vi "Center Spin FR.vi"(0 "Wanted Angle":dbl, 1 "Current Angle":dbl) -> (7 "Motor Output":dbl format="%#_13g")   [LabVIEW 2020]
uses:
  <vilib>/addons/control/pid/pid.llb/PID (DBL).vi
  <vilib>/addons/control/pid/NI_PID_pid.lvlib
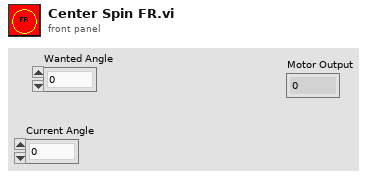
[diagram p1: front panel]
types:
  T1 = cluster{"proportional gain (Kc)":dbl, "integral time (Ti, min)":dbl, "derivative time (Td, min)":dbl}
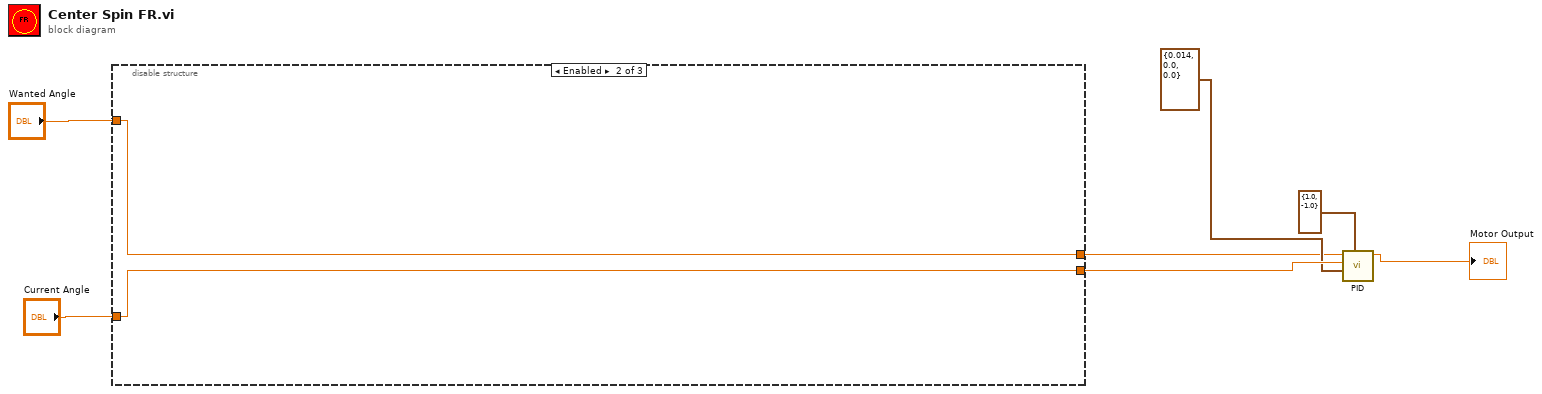
[diagram p0: block diagram]
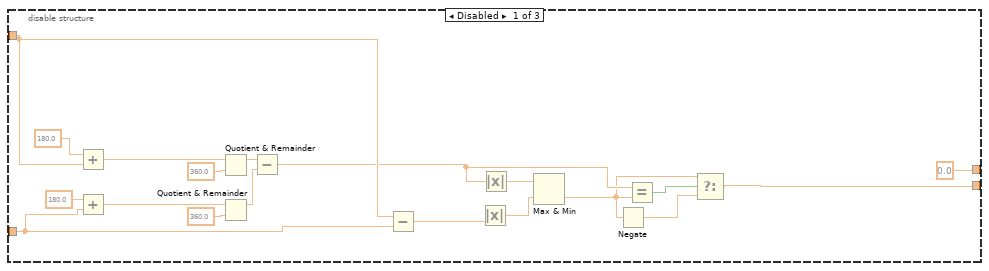
[diagram p2: hidden frame]
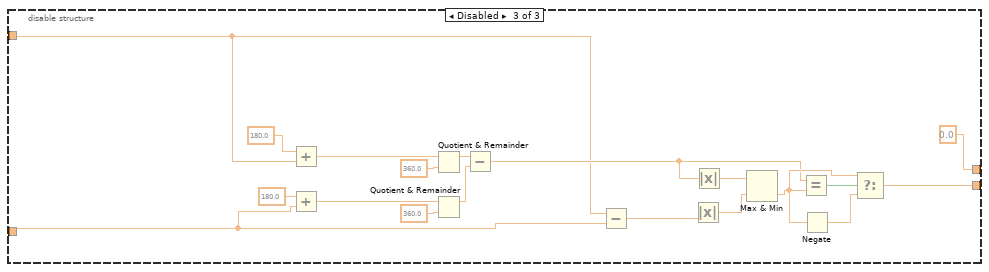
[diagram p3: hidden frame]
diagram:
  n1 = disable-structure shown="Enabled" {
    disable-tunnel: "Current Angle" -> [w26 w27 w31]
    disable-tunnel: "Wanted Angle" -> [w25 w28 w32]
    disable-tunnel: [w24 w27 w30] -> w4
    disable-tunnel: [0.0 w28 0.0] -> w1
    frame Disabled {
      n2 = Add(x=180.0, y=w25) -> (x+y=w10:dbl)
      n3 = Add(x=180.0, y=w26) -> (x+y=w11:dbl)
      n4 = Quotient & Remainder(x=w10, y=360.0) -> (x-y*floor(x/y)=w17:dbl)  [unwired: 1 out]
      n5 = Quotient & Remainder(x=w11, y=360.0) -> (x-y*floor(x/y)=w16:dbl)  [unwired: 1 out]
      n6 = Subtract(x=w17, y=w16) -> (x-y=w15:dbl)
      n7 = Subtract(x=w25, y=w26) -> (x-y=w18:dbl)
      n8 = Absolute Value(x=w18) -> (abs(x)=w12:dbl)
      n9 = Absolute Value(x=w15) -> (abs(x)=w9:dbl)
      n10 = Max & Min(x=w9, y=w12) -> (min(x,y)=w13:dbl)  [unwired: 1 out]
      n11 = Negate(x=w13) -> (-x=w14:dbl)
      n12 = Equal?(x=w15, y=w13) -> (x = y?=w23:bool)
      n13 = Select(t=w13, s=w23, f=w14) -> (s? t:f=w24:dbl)
    }
    frame Enabled {
    }
    frame Disabled {
      n14 = Add(x=180.0, y=w32) -> (x+y=w40:dbl)
      n15 = Add(x=180.0, y=w31) -> (x+y=w41:dbl)
      n16 = Quotient & Remainder(x=w40, y=360.0) -> (x-y*floor(x/y)=w43:dbl)  [unwired: 1 out]
      n17 = Quotient & Remainder(x=w41, y=360.0) -> (x-y*floor(x/y)=w42:dbl)  [unwired: 1 out]
      n18 = Subtract(x=w43, y=w42) -> (x-y=w33:dbl)
      n19 = Subtract(x=w32, y=w31) -> (x-y=w36:dbl)
      n20 = Absolute Value(x=w36) -> (abs(x)=w39:dbl)
      n21 = Absolute Value(x=w33) -> (abs(x)=w37:dbl)
      n22 = Max & Min(x=w37, y=w39) -> (min(x,y)=w35:dbl)  [unwired: 1 out]
      n23 = Equal?(x=w33, y=w35) -> (x = y?=w38:bool)
      n24 = Negate(x=w35) -> (-x=w34:dbl)
      n25 = Select(t=w35, s=w38, f=w34) -> (s? t:f=w30:dbl)
    }
  }
  n26 = call-poly <vilib>:"PID.vi"("output range"=cluster{"output high":dbl, "output low":dbl} {"output high"=1.0, "output low"=-1.0}, "PID gains"=T1 {"proportional gain (Kc)"=0.014, "integral time (Ti, min)"=0.0, "derivative time (Td, min)"=0.0} ("FR Pivot Motor PID gains"), "process variable"=w4, "setpoint"=w1) -> ("output"=→"Motor Output":dbl)  [unwired: 6 in, 1 out]
